vi "Table Name.vi"(11 "Entity in":refnum<class "Entity.lvclass">) -> (2 "Table Name":string, 3 "Entity out":refnum<class "Entity.lvclass">)   [LabVIEW 2022 SP3, in "Conditum.lvlib" / "Entity.lvclass"]
uses:
  Entity.lvclass
  <vilib>/regexp/Match Regular Expression.xnode
  Entity.lvclass/Entity.ctl
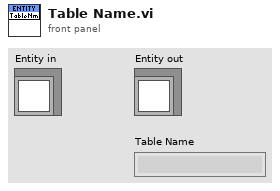
[diagram p1: front panel]
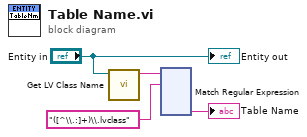
[diagram p0: block diagram]
diagram:
  n1 = call <vilib>:"Get LV Class Name.vi"("object"="Entity in") -> ("class name"=w3:string)  [unwired: 9 in, 1 out]
  n2 = xnode "Match Regular Expression"("input string"=w3, "regular expression"="([^\\.:]+)\\.lvclass") -> ("submatch 1"=→"Table Name":string)  [unwired: 4 in, 5 out]
  "Entity out" <- "Entity in"
